vi "get info from tree tag data.vi"(8 "error in (no error)":errorcluster, 11 "NewVal":string) -> (0 "error out":errorcluster, 2 "item name":string, 3 "CD ref":T1 format="%.0x")   [LabVIEW 2016, in "FPGA RM System Definition API.lvlib"]
doc: "the single page tree control store config info as json in its tag. This unflattens that json and returns it."
uses:
  FPGA RM System Definition API.lvlib
  <vilib>/NI Veristand/Custom Device API/Custom Device Item Ref.ctl
  <vilib>/NI VeriStand/Custom Device API/Custom Device API.lvlib
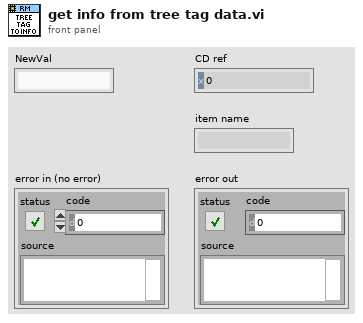
[diagram p1: front panel]
types:
  T1 = typedef "Custom Device API.lvlib/Custom Device Item Ref.ctl" = u64
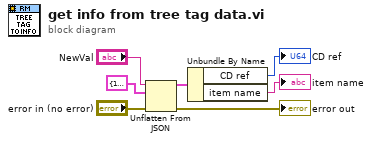
[diagram p0: block diagram]
diagram:
  n1 = Unflatten From JSON(JSON string="NewVal", type and defaults=cluster{"CD ref":T1, "item name":string} {"CD ref"=18446744073709551615, "item name"=""}, error in (no error)="error in (no error)") -> (value=w5:cluster{"CD ref":T1, "item name":string}, error out=→"error out":errorcluster)  [unwired: 4 in]
  n2 = Unbundle By Name(w5) -> ("CD ref"=→"CD ref":T1, "item name"=→"item name":string)
